vi "Item to Name.vi"(11 "Item in":T1) -> (2 "Display Name":string, 3 "Item out":T1)   [LabVIEW 2015, in "Read-Write-Signals.xnode"]
uses:
  Read-Write-Signals.xnode
  Read-Write-Signals Item.ctl
  Read-Write-Signals Sub Item.ctl
  Read-Write-Signals Sub Item Type.ctl
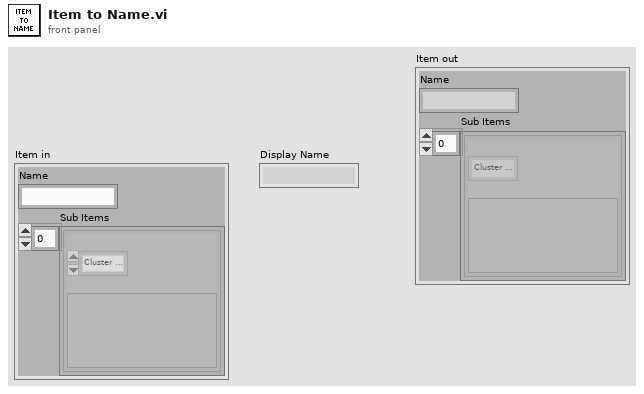
[diagram p1: front panel]
types:
  T1 = typedef "Read-Write-Signals Item.ctl" = cluster{"Name":string, "Sub Items":T2[]}
  T2 = typedef "Read-Write-Signals Sub Item.ctl" = cluster{"Type":T3, "Value":variant}
  T3 = typedef "Read-Write-Signals Sub Item Type.ctl" = enum8{"Cluster Element", "Array Element", "Subarray"}
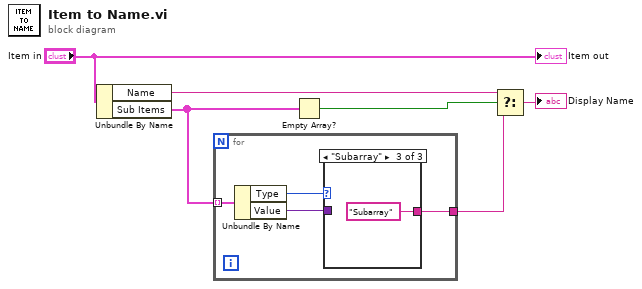
[diagram p0: block diagram]
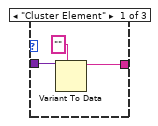
[diagram p2: hidden frame]
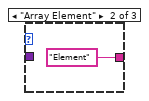
[diagram p3: hidden frame]
diagram:
  n1 = Unbundle By Name("Item in") -> ("Name"=w4:string, "Sub Items"=w6:T2[])
  n2 = for {
    tunnel: w6 -> [w10] mode=indexing
    tunnel: [w7] -> w3
    n3 = Unbundle By Name(w10) -> ("Type"=w8:T3, "Value"=w9:variant)
    n4 = case shown="\"Subarray\"" w8 {
      tunnel: w9 -> [w13 _ _]
      tunnel: [w11 "Element" "Subarray"] -> w7
      frame "Cluster Element" {
        n5 = Variant To Data(type="", Variant=w13) -> (data=w11:string)  [unwired: 1 in, 1 out]
      }
      frame "Array Element" {
      }
      frame "Subarray" {
      }
    }
  }
  n6 = Empty Array?(array=w6) -> (empty?=w5:bool)
  n7 = Select(t=w4, s=w5, f=w3) -> (s? t:f=→"Display Name":string)
  "Item out" <- "Item in"
